vi "Sting Pot Value.vi"() -> ()   [LabVIEW 2013]
panel:
  out "Pot Voltage":dbl
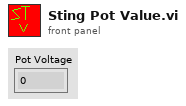
[diagram p1: front panel]
diagram:
